vi "FTS GetSet Acquisition Option AttenuatorAuto.vi"(0 "spectrIdx":u16, 5 "channel":u16, 7 "attenuator auto":bool, 12 "readWrite":enum16{"read", "write"}(ring)) -> (4 "FTSLib status":i32, 8 "auto read":bool)   [LabVIEW 2010, in "FTSLib.lvlib"]
uses:
  FTSLib.lvlib
  FTSLib.dll
panel:
  out "filterStatus_write":u16 format="%04b"
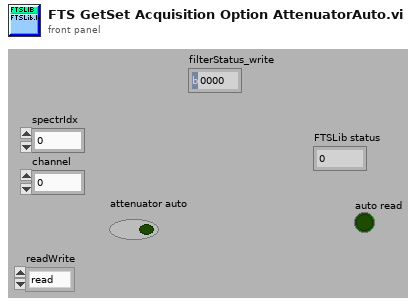
[diagram p1: front panel]
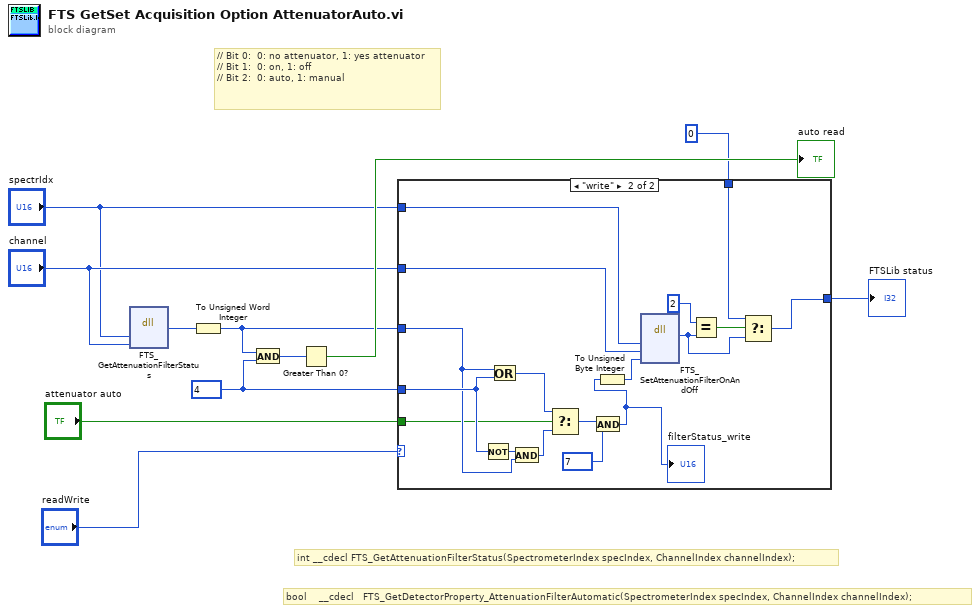
[diagram p0: block diagram]
diagram:
  w5 = u16 4 ("return type")
  # "// Bit 0:  0: no attenuator, 1: yes attenuator\n// Bit 1:  0: on, 1: off\n// Bit 2:  0: auto, 1: manual"
  # "int __cdecl FTS_GetAttenuationFilterStatus(SpectrometerIndex specIndex, ChannelIndex channelIndex);"
  # "bool \t\t\t__cdecl   FTS_GetDetectorProperty_AttenuationFilterAutomatic(SpectrometerIndex specIndex, ChannelIndex channelIndex);"
  n1 = dll-call lib="FTSLib.dll" fn="FTS_GetAttenuationFilterStatus"("spectrIdx"="spectrIdx", "channel"="channel") -> ("return type"=w11:i32)  [unwired: 5 in, 2 out]
  n2 = To Unsigned Word Integer(number=w11) -> (unsigned 16bit integer=w7:u16)
  n3 = And(x=w7, y=w5) -> (x .and. y?=w10:u16)
  n4 = Greater Than 0?(x=w10) -> (x > 0?=→"auto read":bool)
  n5 = case shown="\"write\"" "readWrite" {
    tunnel: w7 -> [_ w20]
    tunnel: "attenuator auto" -> [_ w18]
    tunnel: w5 -> [_ w26]
    tunnel: "channel" -> [_ w28]
    tunnel: "spectrIdx" -> [_ w27]
    tunnel: [w12 w16] -> w2
    tunnel: 0 ("return type") -> [w12 w17]
    frame "read", Default {
    }
    frame "write" {
      n6 = Not(x=w26) -> (.not. x?=w25:u16)
      n7 = Or(x=w20, y=w26) -> (x .or. y?=w19:u16)
      n8 = And(x=w25, y=w20) -> (x .and. y?=w24:u16)
      n9 = Select(t=w19, s=w18, f=w24) -> (s? t:f=w23:u16)
      n10 = And(x=w23, y=u16 7 ("return type")) -> (x .and. y?=w21:u16)
      "filterStatus_write" <- w21
      n11 = To Unsigned Byte Integer(number=w21) -> (unsigned 8bit integer=w29:u8)
      n12 = dll-call lib="FTSLib.dll" fn="FTS_SetAttenuationFilterOnAndOff"("spectrIdx"=w27, "channel"=w28, "filterStatus"=w29) -> ("return type"=w13:i32)  [unwired: 6 in, 2 out]
      n13 = Equal?(x=2, y=w13) -> (x = y?=w14:bool)
      n14 = Select(t=w17, s=w14, f=w13) -> (s? t:f=w16:i32)
    }
  }
  "FTSLib status" <- w2
